vi "Rx DUT Command.vi"(8 "error in (no error)":errorcluster, 11 "DUT Sample in":refnum<class "DUT Sample.lvclass">) -> (0 "error out":errorcluster, 2 "Commands":T1[](array[typedef]), 3 "DUT Sample out":refnum<class "DUT Sample.lvclass">)   [LabVIEW 2023, in "DUT Sample.lvclass"]
uses:
  DUT Sample.lvclass
  DUT Sample.lvclass/DUT Sample.ctl
  typedefs/DUT Command Type.ctl
  typedefs/DUT Command.ctl
  <vilib>/xnet/xnet.llb/XNET Read (Signal Single-point).vi
  typedefs/DO Finite Pulse Config.ctl
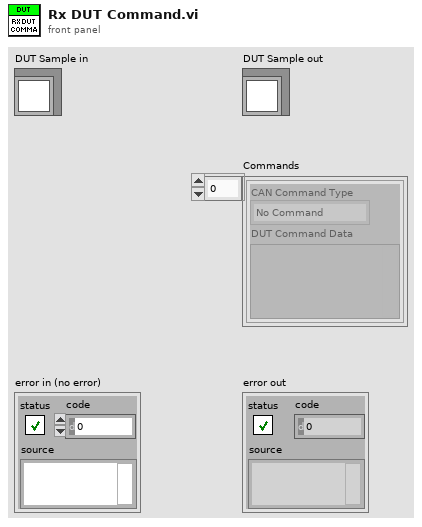
[diagram p1: front panel]
types:
  T1 = typedef "DUT Sample.lvclass/DUT Command.ctl" = cluster{"CAN Command Type":T2, "DUT Command Data":variant}
  T2 = typedef "DUT Sample.lvclass/DUT Command Type.ctl" = enum16{"No Command", "Generate DO Pulse"}
  T3 = typedef "DUT Sample.lvclass/DO Finite Pulse Config.ctl" = cluster{"Port Number":u8, "Number of Pulses":u8, "High Time (ms)":u16, "Low Time (ms)":u16}
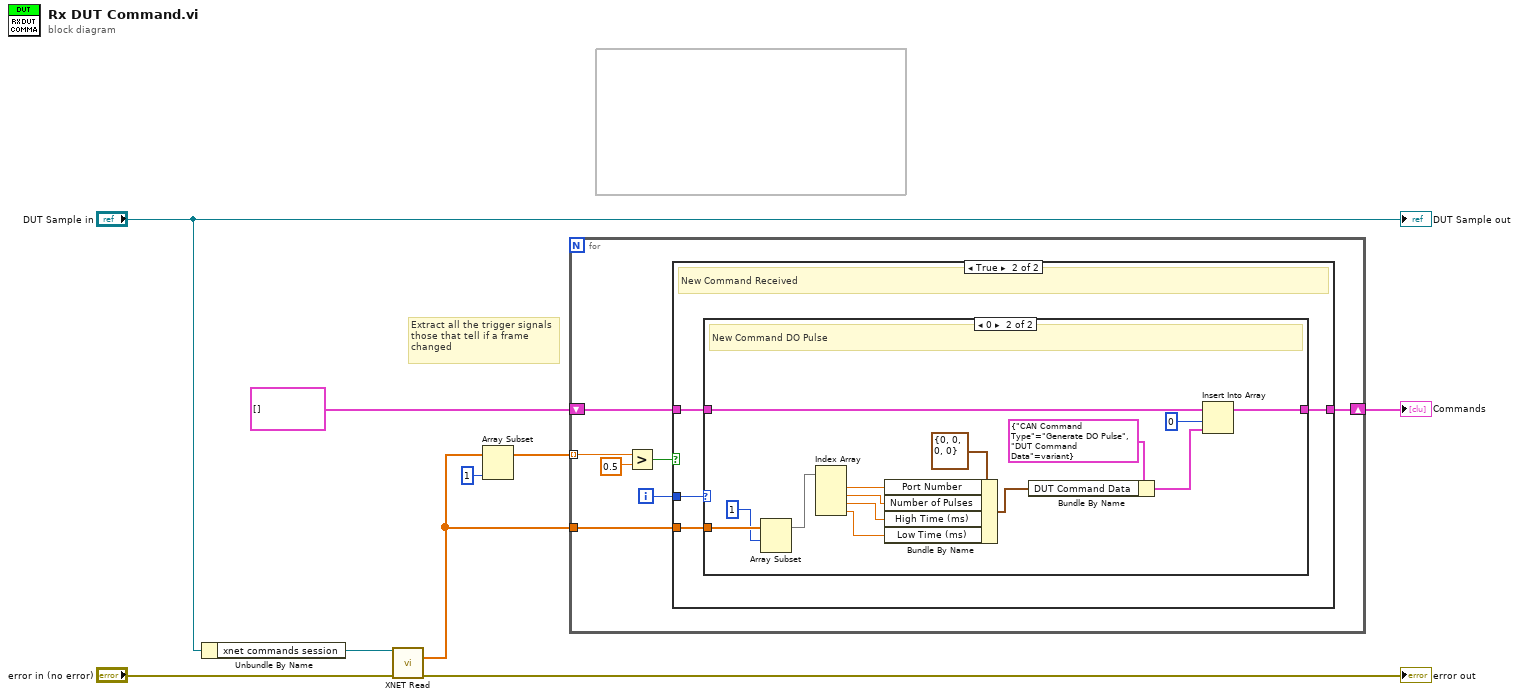
[diagram p0: block diagram]
diagram:
  # "Extract all the trigger signals\nthose that tell if a frame\nchanged"
  n1 = Unbundle By Name("DUT Sample in") -> ("xnet commands session"=w6:refnum<k21>)
  n2 = call-poly <vilib>:"XNET Read.vi"("session in"=w6, "error in (no error)"="error in (no error)") -> ("data"=w1:dbl[], "error out"=→"error out":errorcluster)  [unwired: 12 out]
  n3 = Array Subset "Array Subset"(array=w1, length=1) -> (w3:dbl[])  [unwired: 1 in]
  n4 = for {
    tunnel: w1 -> [w15]
    tunnel: w3 -> [w12] mode=indexing
    shift-right: [w13] -> w4
    shift-left: T1[] [] ("CAN Commands") -> [w14]
    i -> [w11]
    n5 = Greater?(x=w12, y=0.5) -> (0:w10:bool)
    n6 = case shown="True" w10 {
      tunnel: w15 -> [_ w21]
      tunnel: w14 -> [w17 w20]
      tunnel: [w17 w19] -> w13
      tunnel: w11 -> [_ w18]
      frame False {
        # "This frame did not change since the last read"
      }
      frame True {
        # "New Command Received"
        n7 = case shown="0" w18 {
          tunnel: w21 -> [_ w30]
          tunnel: w20 -> [w22 w33]
          tunnel: [w22 w32] -> w19
          frame Default {
            # "Unknown command"
          }
          frame 0 {
            # "New Command DO Pulse"
            n8 = Array Subset(array=w30, index=1) -> (w24:dbl[])  [unwired: 1 in]
            n9 = Index Array(array=w24) -> (element #1=w28:dbl, element #2=w27:dbl, element #3=w26:dbl, element #4=w29:dbl)  [unwired: 4 in]
            n10 = Bundle By Name(cluster=T3 {"Port Number"=0, "Number of Pulses"=0, "High Time (ms)"=0, "Low Time (ms)"=0} ("DO Finite Pulse Config"), "Port Number"=w28, "Number of Pulses"=w27, "High Time (ms)"=w26, "Low Time (ms)"=w29) -> (w25:T3)
            n11 = Bundle By Name(cluster=T1 {"CAN Command Type"=enum."Generate DO Pulse", "DUT Command Data"=variant} ("CAN Command"), "DUT Command Data"=w25) -> (w34:T1)
            n12 = Insert Into Array "Insert Into Array"(array=w33, index=0, new element=w34) -> (w32:T1[])
          }
        }
      }
    }
  }
  "Commands" <- w4
  "DUT Sample out" <- "DUT Sample in"
